vi "Files for Active Electrode.vi"(6 "error in":errorcluster, 9 "index":i32) -> (0 "error out":errorcluster={"status"=TRUE, "code"=43, "source"="File Dialog"}, 1 "Average Size":dbl=15.0, 2 "Resistance (ohms)":dbl format="%.1f", 3 "WaveformP":waveform(dbl)(graph), 4 "Filename":path)   [LabVIEW 2010]
panel:
  in  "Rmeas (ohms)":dbl[](array[numeric])=[500.0, 10000.0, 500.0, 500.0, 10000.0, 500.0, 500.0, 500.0]
  in  "Data Files":path[](array[path])=[path "C:/5-01-003 Active Electrode Min Max/Post Differential Waveform 1 -5 mA", path "C:/5-01-003 Active Electrode Min Max/Post Differential Waveform 2 -0.02 mA", path "C:/5-01-003 Active Electrode Min Max/Post Differential Waveform 3 -15 mA", path "C:/5-01-003 Active Electrode Min Max/Post Differential Waveform 4 3 mA", path "C:/5-01-003 Active Electrode Min Max/Post Differential Waveform 5 0.02 mA", path "C:/5-01-003 Active Electrode Min Max/Post Differential Waveform 6 15 mA", path "", path ""]
  out "Waveform":waveform(dbl)={"t0"=timestamp(0 s since 1904-01-01), "dt"=nan, "Y"=[]}
  # "0"
  # "1"
  # "2"
  # "3"
  # "4"
  # "5"
  # "6"
  # "7"
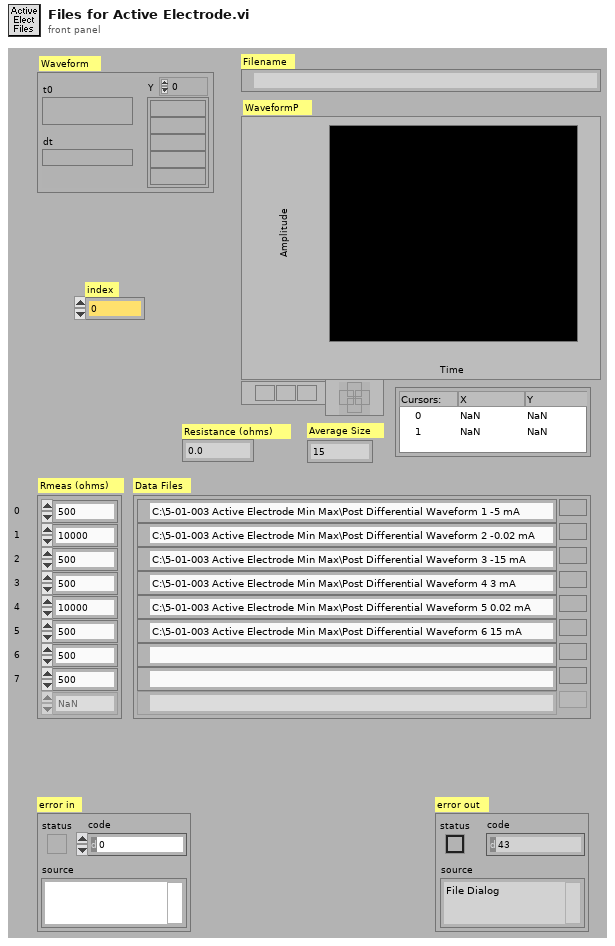
[diagram p1: front panel]
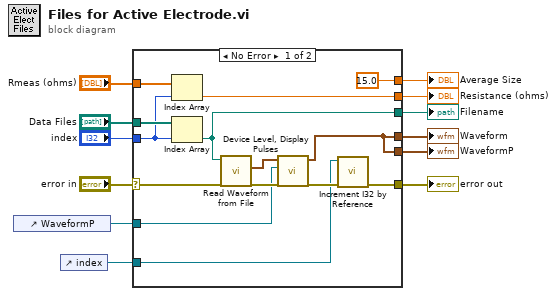
[diagram p0: block diagram]
diagram:
  n1 = control-ref of="WaveformP"() -> (w2:refnum<vi>)
  n2 = control-ref of="index"() -> (w1:refnum<vi>)
  n3 = case shown="No Error" "error in" {
    selector: "error in" -> [w26 w27]
    tunnel: [w14 w27] -> w8
    tunnel: "Data Files" -> [w25 _]
    tunnel: "index" -> [w23 _]
    tunnel: "Rmeas (ohms)" -> [w24 _]
    tunnel: [w16 _] -> w7
    tunnel: [w16 _] -> w6
    tunnel: [w22 _] -> w5
    tunnel: [15.0 ("Num") _] -> w4
    tunnel: [w20 _] -> w3
    tunnel: w2 -> [w17 _]
    tunnel: w1 -> [w13 _]
    frame No Error {
      n4 = Index Array(array=w24, index=w23) -> (element=w22:dbl)
      n5 = Index Array(array=w25, index=w23) -> (element=w20:path)
      n6 = call <vilib>:"Read Waveform from File.vi"("error in (no error)"=w26, "file path (dialog if empty)"=w20) -> ("error out"=w19:errorcluster, "first waveform in record"=w18:waveform(dbl))  [unwired: 4 in, 2 out]
      n7 = call "Device Level, Display Pulses.vi"("error in"=w19, "WFGraph Refnum"=w17, "waveform"=w18) -> ("error out"=w15:errorcluster, "waveform dup"=w16:waveform(dbl))  [unwired: 6 in]
      n8 = call "Increment I32 by Reference.vi"("error in"=w15, "dignum refnum"=w13) -> ("error out"=w14:errorcluster)  [unwired: 6 in, 2 out]
    }
    frame Error {
    }
  }
  "Average Size" <- w4
  "error out" <- w8
  "WaveformP" <- w7
  "Waveform" <- w6
  "Resistance (ohms)" <- w5
  "Filename" <- w3
